vi "Ask_640_power.vi"(8 "error in":errorcluster, 11 "VISA resource name":refnum<visa-resource-name>) -> (0 "error out":errorcluster, 2 "640 Power":dbl, 3 "VISA resource name out":refnum<visa-resource-name>)   [LabVIEW 2015]
panel:
  out "Serial Settings:Number of Bytes at Serial Port":u32
  out "read buffer":string
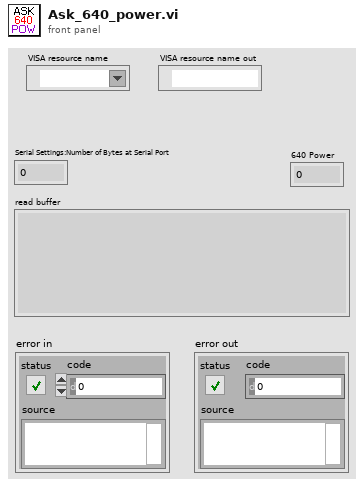
[diagram p1: front panel]
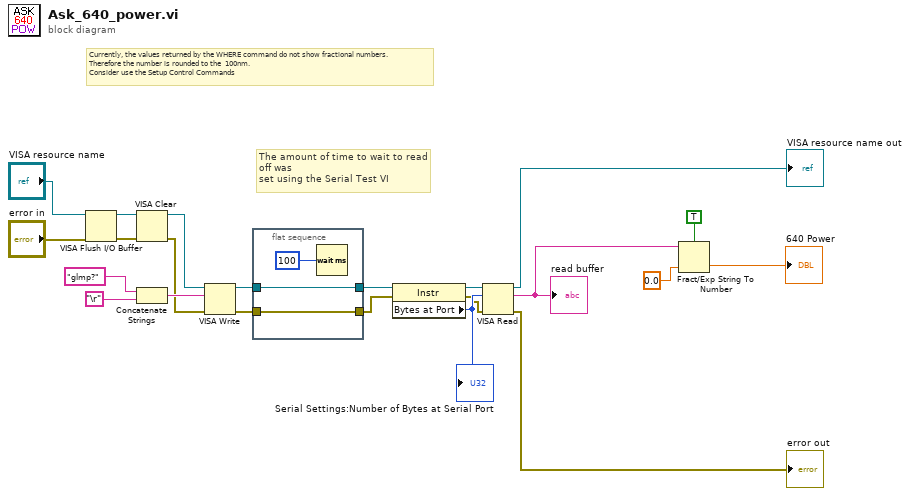
[diagram p0: block diagram]
diagram:
  # "Currently, the values returned by the WHERE command do not show fractional numbers.\nTherefore the number is rounded to the  100nm. \nConsider use the Setup Control Commands"
  # "The amount of time to wait to read off was \nset using the Serial Test VI"
  n1 = VISA Flush I/O Buffer(VISA resource name="VISA resource name", error in (no error)="error in") -> (VISA resource name out=w3:refnum<visa-resource-name>, error out=w1:errorcluster)  [unwired: 1 in]
  n2 = VISA Clear(VISA resource name=w3, error in (no error)=w1) -> (VISA resource name out=w6:refnum<visa-resource-name>, error out=w5:errorcluster)
  n3 = Concatenate Strings("glmp?" ("string"), "\r") -> (w13:string)
  n4 = VISA Write(VISA resource name=w6, write buffer=w13, error in (no error)=w5) -> (VISA resource name out=w19:refnum<visa-resource-name>, error out=w17:errorcluster)  [unwired: 1 out]
  n5 = flat-sequence {
    tunnel: [w25] -> w20
    tunnel: w19 -> [w25]
    tunnel: [w23] -> w18
    tunnel: w17 -> [w23]
    frame #0 {
      n6 = Wait (ms)(milliseconds to wait=u32 100) -> ()  [unwired: 1 out]
    }
  }
  n7 = property class="Instr"(reference=w20, error in=w18) -> (reference out=w22:refnum<visa-resource-name>, error out=w16:errorcluster, "Bytes at Port"=w21:u32)
  "Serial Settings:Number of Bytes at Serial Port" <- w21
  n8 = VISA Read(VISA resource name=w22, byte count=w21, error in (no error)=w16) -> (VISA resource name out=→"VISA resource name out":refnum<visa-resource-name>, read buffer=w8:string, error out=→"error out":errorcluster)  [unwired: 1 out]
  "read buffer" <- w8
  n9 = Fract/Exp String To Number(use system decimal point (T)=TRUE, string=w8, default (0 dbl)=0.0 ("default (0 I32)")) -> (number=→"640 Power":dbl)  [unwired: 1 in, 1 out]
